vi "build-island-msg.vi"(4 "error (in)":errorcluster, 5 "base":cluster{"type":dbl, "mode":dbl, "sequence":dbl}, 6 "param":T1, 7 "change-mode-to":string(combo)) -> (0 "error (out)":errorcluster, 3 "JSON string":string)   [LabVIEW 2021]
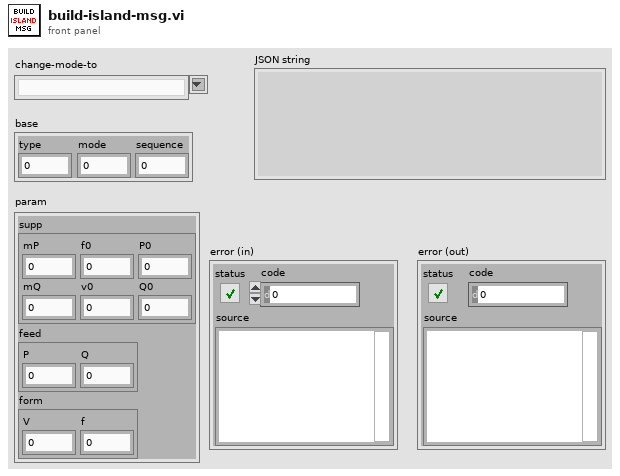
[diagram p1: front panel]
types:
  T1 = cluster{"supp":cluster{"mP":dbl, "f0":dbl, "P0":dbl, "v0":dbl, "mQ":dbl, "Q0":dbl}, "form":cluster{"V":dbl, "f":dbl}, "feed":cluster{"P":dbl, "Q":dbl}}
  T2 = cluster{"parameters":cluster{"mP":dbl, "f0":dbl, "P0":dbl, "v0":dbl, "mQ":dbl, "Q0":dbl}, "mode":dbl, "type":dbl, "sequence":dbl}
  T3 = cluster{"parameters":cluster{"P":dbl, "Q":dbl}, "mode":dbl, "type":dbl, "sequence":dbl}
  T4 = cluster{"parameters":cluster{"V":dbl, "f":dbl}, "mode":dbl, "type":dbl, "sequence":dbl}
  T5 = cluster{"mP":dbl, "f0":dbl, "P0":dbl, "v0":dbl, "mQ":dbl, "Q0":dbl}
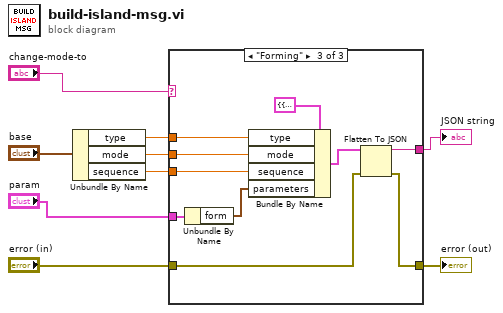
[diagram p0: block diagram]
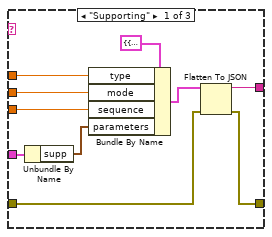
[diagram p2: hidden frame]
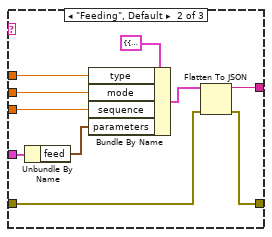
[diagram p3: hidden frame]
diagram:
  n1 = Unbundle By Name("base") -> ("type"=w6:dbl, "mode"=w5:dbl, "sequence"=w4:dbl)
  n2 = case shown="\"Forming\"" "change-mode-to" {
    tunnel: "param" -> [w19 w29 w39]
    tunnel: w6 -> [w17 w26 w37]
    tunnel: w5 -> [w16 w25 w36]
    tunnel: w4 -> [w15 w24 w35]
    tunnel: [w12 w22 w32] -> w3
    tunnel: "error (in)" -> [w11 w21 w30]
    tunnel: [w10 w20 w31] -> w1
    frame "Supporting" {
      n3 = Unbundle By Name(w19) -> ("supp"=w14:T5)
      n4 = Bundle By Name(cluster=T2 {"parameters"={"mP"=0.0, "f0"=0.0, "P0"=0.0, "v0"=0.0, "mQ"=0.0, "Q0"=0.0}, "mode"=0.0, "type"=0.0, "sequence"=0.0} ("supp"), "type"=w17, "mode"=w16, "sequence"=w15, "parameters"=w14) -> (w13:T2)
      n5 = Flatten To JSON(anything=w13, error in (no error)=w11) -> (JSON string=w12:string, 11:w10:errorcluster)  [unwired: 1 in]
    }
    frame "Feeding", Default {
      n6 = Unbundle By Name(w29) -> ("feed"=w27:cluster{"P":dbl, "Q":dbl})
      n7 = Bundle By Name(cluster=T3 {"parameters"={"P"=0.0, "Q"=0.0}, "mode"=0.0, "type"=0.0, "sequence"=0.0} ("feed"), "type"=w26, "mode"=w25, "sequence"=w24, "parameters"=w27) -> (w23:T3)
      n8 = Flatten To JSON(anything=w23, error in (no error)=w21) -> (JSON string=w22:string, 11:w20:errorcluster)  [unwired: 1 in]
    }
    frame "Forming" {
      n9 = Unbundle By Name(w39) -> ("form"=w34:cluster{"V":dbl, "f":dbl})
      n10 = Bundle By Name(cluster=T4 {"parameters"={"V"=0.0, "f"=0.0}, "mode"=0.0, "type"=0.0, "sequence"=0.0} ("form"), "type"=w37, "mode"=w36, "sequence"=w35, "parameters"=w34) -> (w33:T4)
      n11 = Flatten To JSON(anything=w33, error in (no error)=w30) -> (JSON string=w32:string, 11:w31:errorcluster)  [unwired: 1 in]
    }
  }
  "JSON string" <- w3
  "error (out)" <- w1
